vi "ImageSaveImage-1D.vi"(8 "error in (no error)":errorcluster, 10 "Save image":bool, 11 "Image in":refnum<class "Image.lvclass">) -> (0 "error out":errorcluster, 3 "Image out":refnum<class "Image.lvclass">)   [LabVIEW 2012, in "Image.lvclass"]
uses:
  classes/Image.lvclass
  classes/Image.lvclass/Image.ctl
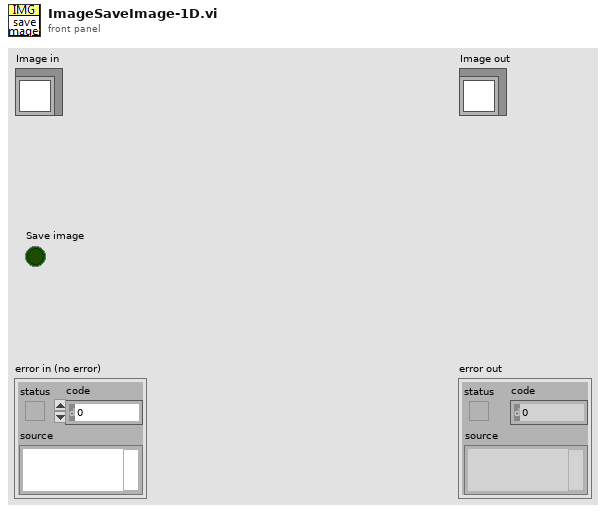
[diagram p1: front panel]
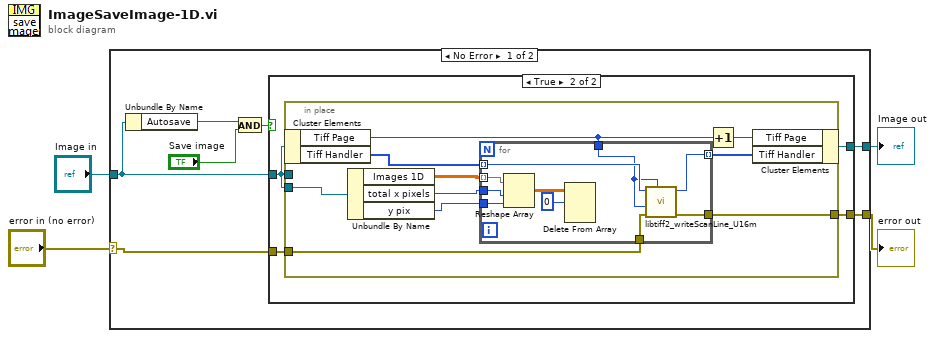
[diagram p0: block diagram]
diagram:
  n1 = case shown="No Error" "error in (no error)" {
    selector: "error in (no error)" -> [w5 _]
    tunnel: [w10 w37] -> w3
    tunnel: "Image in" -> [w11 w37]
    tunnel: [w6 _] -> w1
    frame No Error {
      n2 = Unbundle By Name(w11) -> ("Autosave"=w8:bool)
      n3 = And(x=w8, y="Save image") -> (x .and. y?=w7:bool)
      n4 = case shown="True" w7 {
        tunnel: w11 -> [w12 w15]
        tunnel: [w12 w16] -> w10
        tunnel: [_ w14] -> w6
        tunnel: w5 -> [_ w13]
        frame False {
        }
        frame True {
          n5 = in-place {
            in-place-border: w15 -> [_]
            in-place-border: w15 -> [w22]
            in-place-border: [w21] -> w14
            in-place-border: w13 -> [w20]
            n6 = in-place-cluster #1(w15) -> ("Tiff Page"=w17:u32, "Tiff Handler"=w19:u32[])
            n7 = Unbundle By Name(w22) -> ("Images 1D"=w23:dbl[][][], "total x pixels"=w24:i32, "y pix"=w25:i32)
            n8 = for {
              tunnel: w23 -> [w36] mode=indexing
              tunnel: w24 -> [w35]
              tunnel: w25 -> [w34]
              tunnel: [w31] -> w21
              tunnel: w20 -> [w30]
              tunnel: w19 -> [w29] mode=indexing
              tunnel: [w28] -> w18 mode=indexing
              tunnel: w17 -> [w27]
              n9 = Reshape Array(w36, w35, w34) -> (w33:dbl[][])
              n10 = Delete From Array(array=w33, length=0) -> ()  [unwired: 2 in, 2 out]
              n11 = call "libtiff2_writeScanLine_U16m.vi"("totalpages"=w27, "error in (no error)"=w30, "page"=w27, "Handle"=w29) -> ("error out"=w31:errorcluster, "Handle out"=w28:i32)  [unwired: 6 in]
            }
            n12 = Increment(x=w17) -> (x+1=w26:u32)
            n13 = in-place-cluster #1("Tiff Page"=w26, "Tiff Handler"=w18) -> (w16:refnum<class "Image.lvclass">)
          }
        }
      }
    }
    frame Error {
    }
  }
  "error out" <- w1
  "Image out" <- w3
